vi "LogEventCore.vi"(8 "error in (no error)":errorcluster, 10 "Event":string, 11 "EventLoggerData in in":T1) -> (0 "error out":errorcluster, 3 "EventLoggerData out":T1)   [LabVIEW 2019, in "EventLogger.lvlib"]
uses:
  EventLogger.lvlib
  Cluster - EventLoggerData.ctl
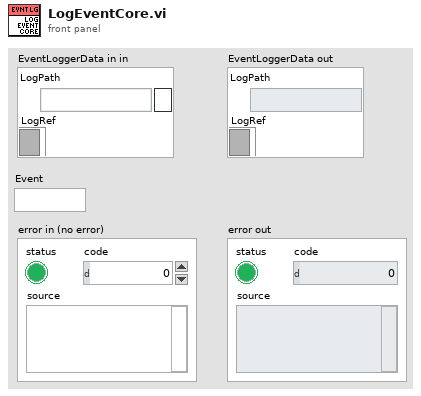
[diagram p1: front panel]
types:
  T1 = typedef "EventLogger.lvlib/Cluster - EventLoggerData.ctl" = cluster{"LogPath":path, "LogRef":refnum<file>}
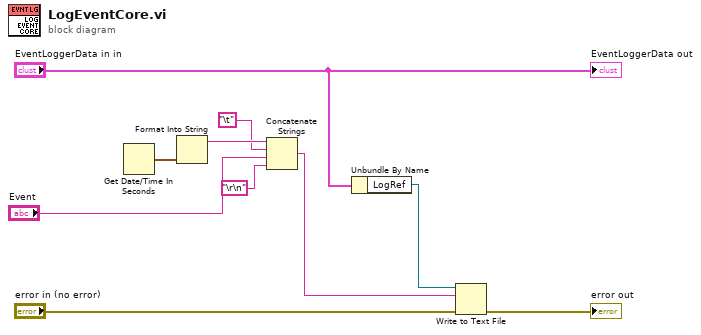
[diagram p0: block diagram]
diagram:
  n1 = Get Date/Time In Seconds() -> (seconds since 1Jan1904=w9:timestamp)
  n2 = Format Into String(w9) -> (resulting string=w8:string)  [unwired: 3 in, 1 out]
  n3 = Concatenate Strings(w8, "\t" ("string"), "Event", "\r\n") -> (w2:string)
  n4 = Unbundle By Name("EventLoggerData in in") -> ("LogRef"=w4:refnum<file>)
  n5 = Write to Text File(file (use dialog)=w4, text=w2, error in="error in (no error)") -> (error out=→"error out":errorcluster)  [unwired: 1 in, 2 out]
  "EventLoggerData out" <- "EventLoggerData in in"
